vi "SPCRatesReady.vi"(1 "Time":u32) -> (0 "Boolean":bool)   [LabVIEW 2009]
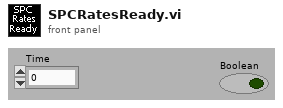
[diagram p1: front panel]
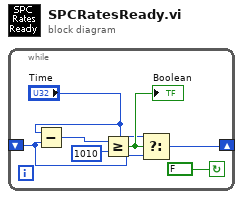
[diagram p0: block diagram]
diagram:
  n1 = while {
    shift-right: [w2] -> _
    shift-left: _ -> [w3]
    stop <- FALSE continue-if-true
    n2 = Subtract(x="Time", y=w3) -> (x-y=w5:u32)
    n3 = Greater Or Equal?(x=w5, y=u32 1010) -> (x >= y?=w7:bool)
    "Boolean" <- w7
    n4 = Select(t="Time", s=w7, f=w3) -> (s? t:f=w2:u32)
  }
